vi "test_BlocRWtest.vi"() -> ()   [LabVIEW 2020]
panel:
  out "size":u64
  out "dst":T1
  out "error out":errorcluster
  out "return":i32
  in  "TY_FDX_UDP_BLOCK_WRITE_IN_MSG":T2(array[cluster])
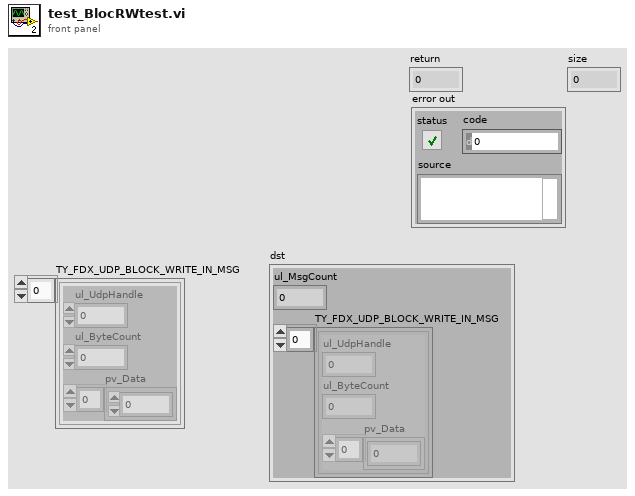
[diagram p1: front panel]
types:
  T1 = cluster{"ul_MsgCount":u32, "TY_FDX_UDP_BLOCK_WRITE_IN_MSG":cluster{"ul_UdpHandle":u32, "ul_ByteCount":u32, "pv_Data":u8[]}[]}
  T2 = cluster{"ul_UdpHandle":u32, "ul_ByteCount":u32, "pv_Data":u8[]}[]
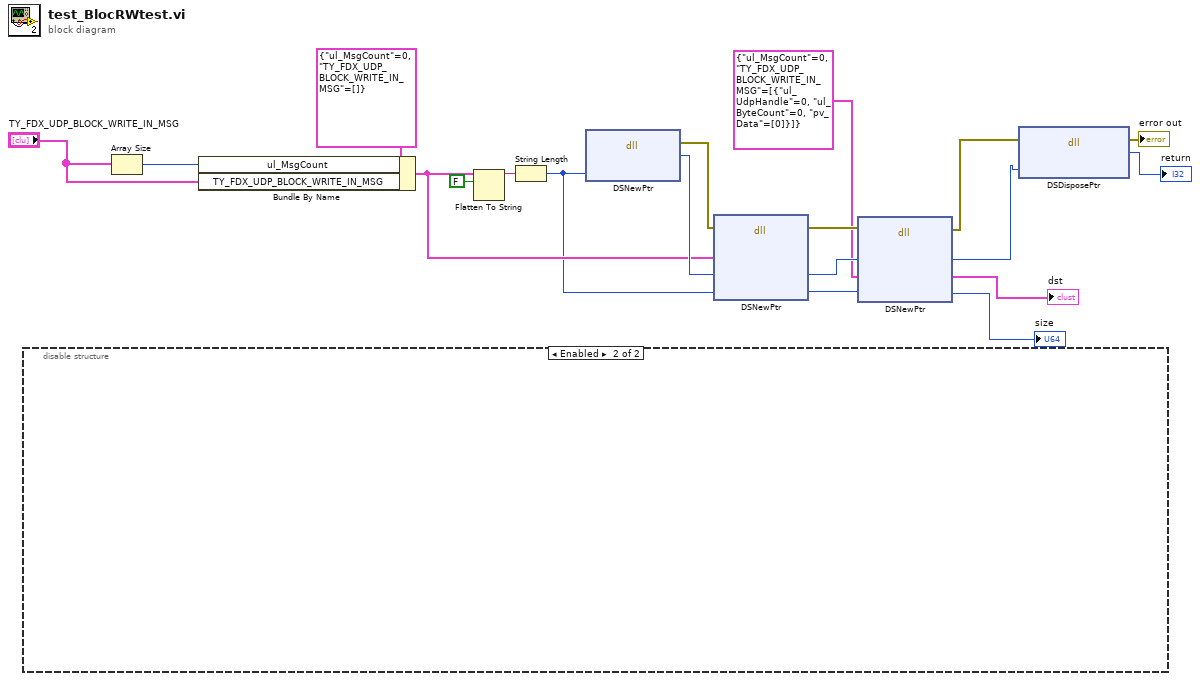
[diagram p0: block diagram]
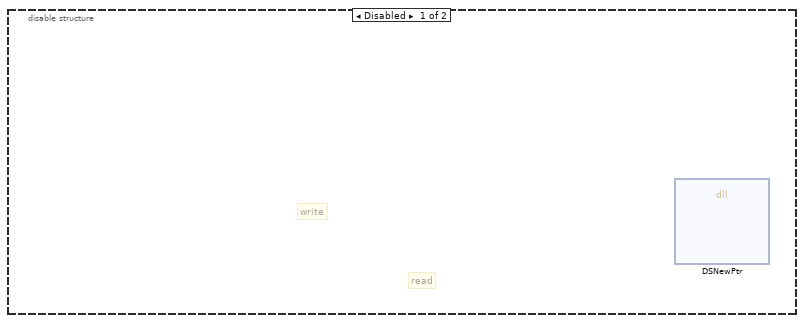
[diagram p2: hidden frame]
diagram:
  n1 = disable-structure shown="Enabled" {
    frame Disabled {
      # "read"
      # "write"
      n2 = dll-call lib="LabVIEW" fn="DSNewPtr"() -> ()  [unwired: 10 in, 2 out]
    }
    frame Enabled {
    }
  }
  n3 = Array Size(array="TY_FDX_UDP_BLOCK_WRITE_IN_MSG") -> (size(s)=w17:i32)
  n4 = Bundle By Name(cluster=T1 {"ul_MsgCount"=0, "TY_FDX_UDP_BLOCK_WRITE_IN_MSG"=[]} ("TY_FDX_UDP_BLOCK_WRITE_IN"), "ul_MsgCount"=w17, "TY_FDX_UDP_BLOCK_WRITE_IN_MSG"="TY_FDX_UDP_BLOCK_WRITE_IN_MSG") -> (w8:T1)
  n5 = Flatten To String(anything=w8, prepend array or string size? (T)=FALSE) -> (data string=w15:string)  [unwired: 2 in, 2 out]
  n6 = String Length(string=w15) -> (length=w7:i32)
  n7 = dll-call lib="LabVIEW" fn="DSNewPtr"("size"=w7) -> (error out=w10:errorcluster, "pointer"=w12:u64)  [unwired: 4 in, 1 out]
  n8 = dll-call lib="LabVIEW" fn="DSNewPtr"(error in=w10, "src"=w8, "dst"=w12, "size"=w7) -> (error out=w9:errorcluster, "dst"=w11:u64, "size"=w6:u64)  [unwired: 4 in, 1 out]
  n9 = dll-call lib="LabVIEW" fn="DSNewPtr"(error in=w9, "src"=w11, "dst"=T1 {"ul_MsgCount"=0, "TY_FDX_UDP_BLOCK_WRITE_IN_MSG"=[{"ul_UdpHandle"=0, "ul_ByteCount"=0, "pv_Data"=[0]}]} ("TY_FDX_UDP_BLOCK_WRITE_IN"), "size"=w6) -> (error out=w1:errorcluster, "src"=w5:u64, "dst"=→"dst":T1, "size"=→"size":u64)  [unwired: 3 in, 1 out]
  n10 = dll-call lib="LabVIEW" fn="DSDisposePtr"(error in=w1, "pointer"=w5) -> (error out=→"error out":errorcluster, "return"=→"return":i32)  [unwired: 3 in, 1 out]
